vi "find_preamble_2x2.vi"(0 "received \ntime symbol":cdb[][](array[numeric]), 5 "FFT Size":u32, 7 "CP Length":u32, 9 "1st preamble":cdb[](array[numeric]), 11 "2nd preamble":cdb[](array[numeric])) -> (4 "Received OFDM symbol (vector)":cdb[](array[numeric]), 6 "Received OFDM symbol (h11)":cdb[](array[numeric]), 8 "Received OFDM symbol (h12)":cdb[](array[numeric]), 10 "Received OFDM symbol (h21)":cdb[](array[numeric]), 15 "Received OFDM symbol (h22)":cdb[](array[numeric]))   [LabVIEW 2020]
uses:
  <vilib>/Analysis/2dsp.llb/2D Complex FFT.vi
  <vilib>/Analysis/baseanly.llb/Complex A x B.vi
  <vilib>/Analysis/baseanly.llb/Complex Inverse Matrix.vi
  <vilib>/Analysis/baseanly.llb/Complex A x Vector.vi
  <vilib>/Analysis/NI_AALBase.lvlib
  <vilib>/Analysis/NI_AALPro.lvlib
panel:
  out "size(s)":i32
  out "Waveform Chart 4":dbl[][](graph)
  out "Array 2":i32[](array[numeric])
  out "x-y 2":i32
  out "max value 4":dbl
  out "max value 3":dbl
  out "Array":i32[](array[numeric])
  out "x-y":i32
  out "max value 2":dbl
  out "max value":dbl
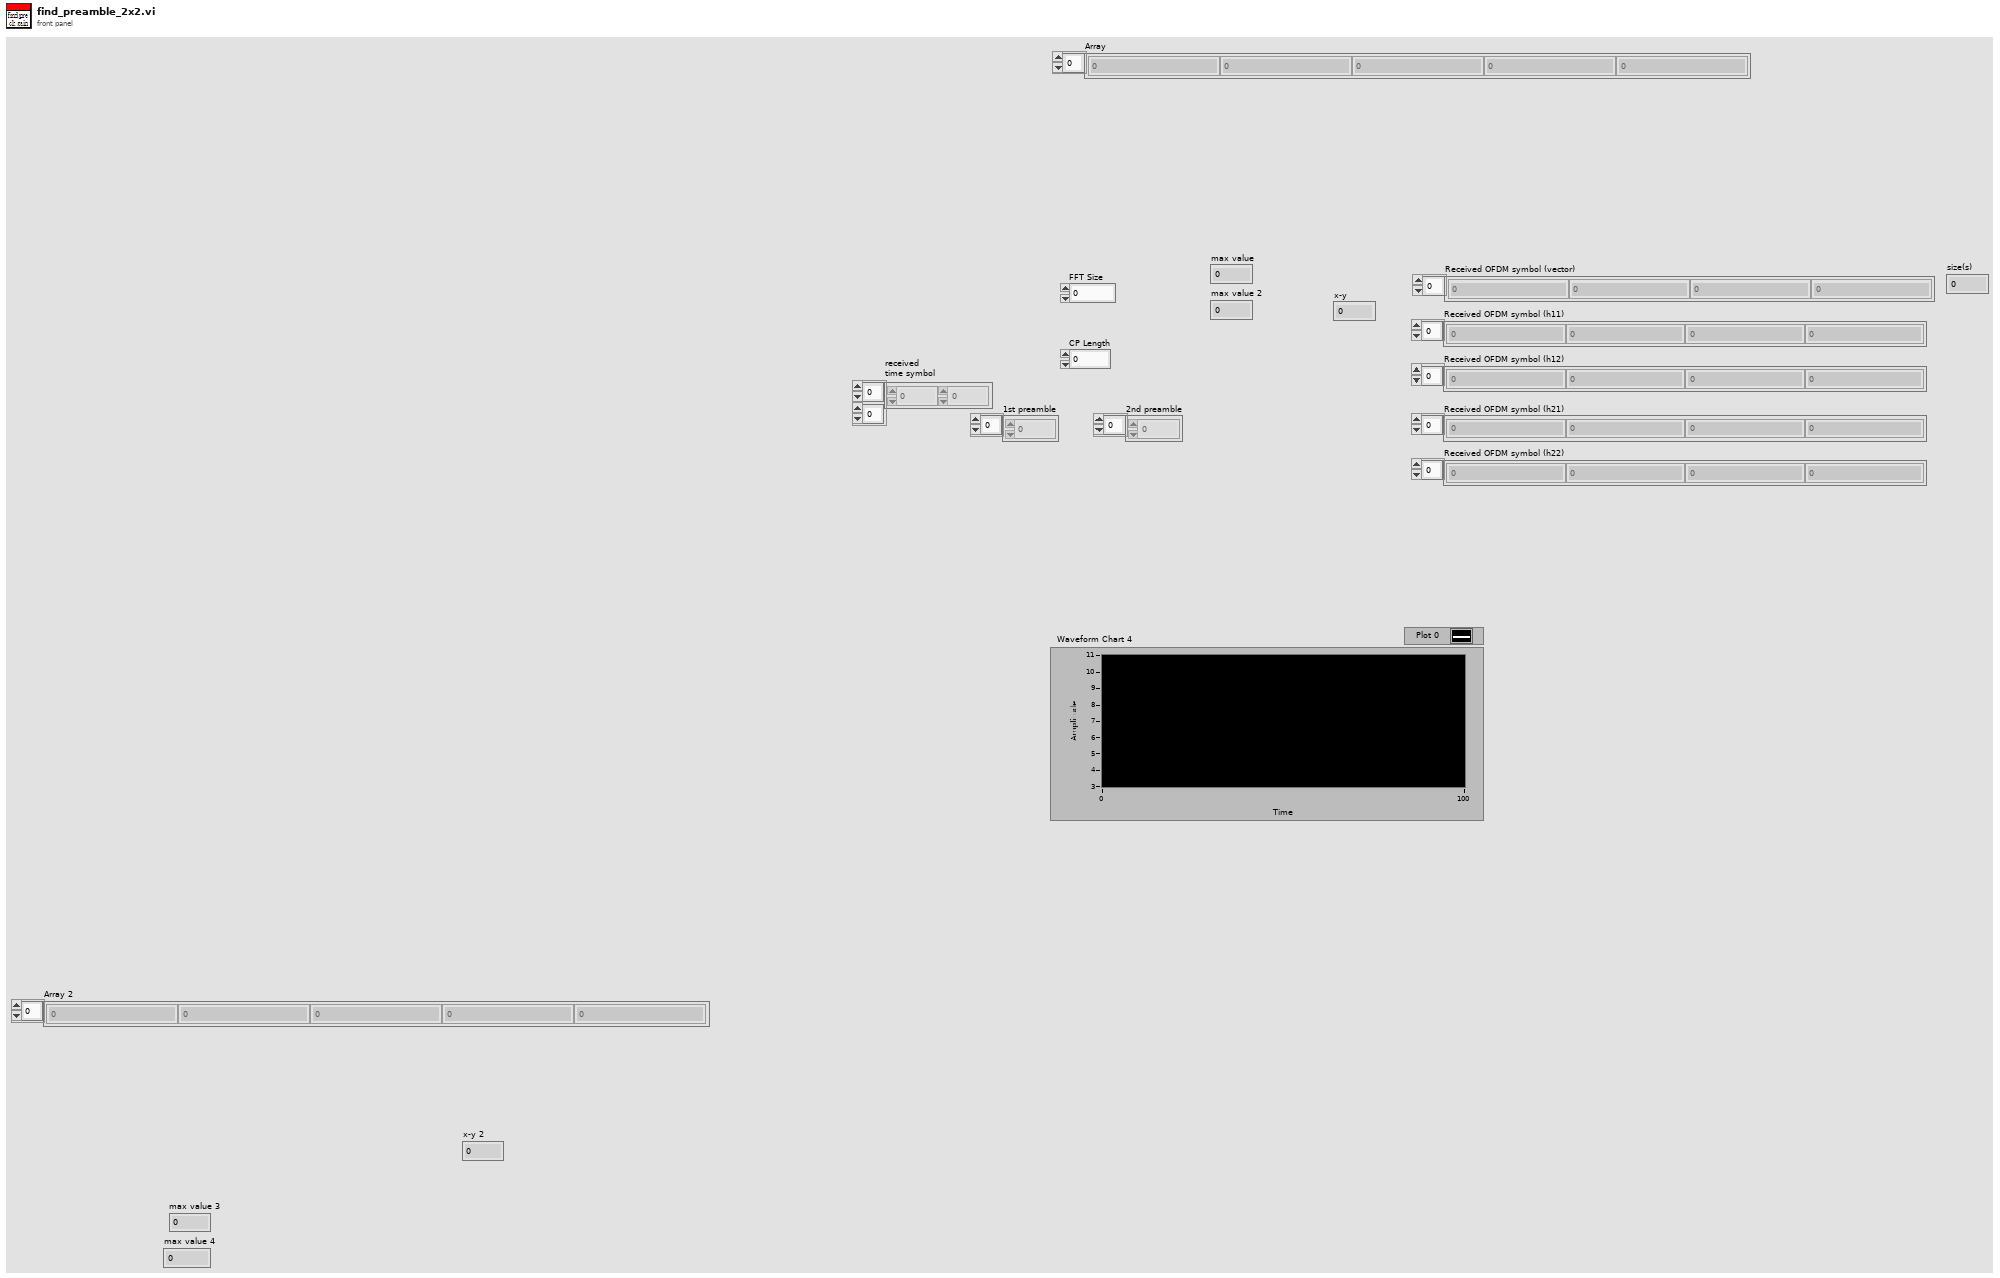
[diagram p1: front panel]
types:
  T1 = typedef "NI_Matrix.lvlib/ComplexMatrix.ctl" = cdb[][]
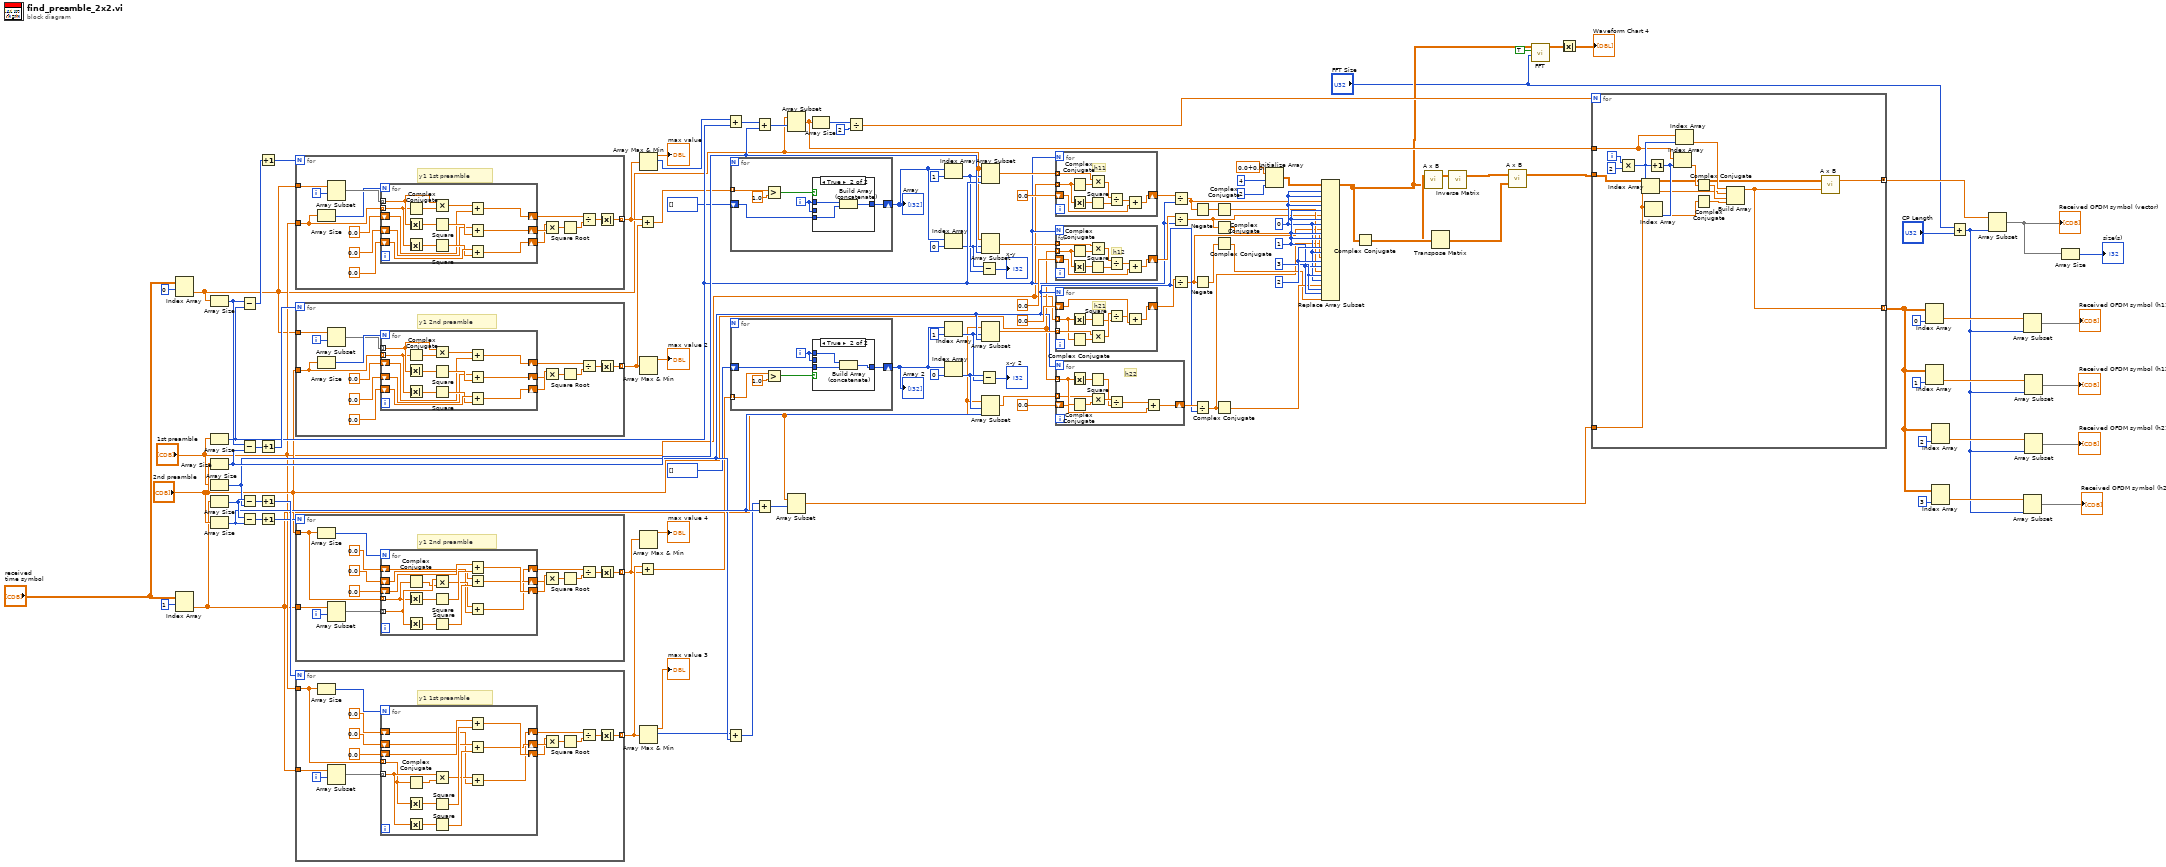
[diagram p0: block diagram]
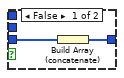
[diagram p2: hidden frame]
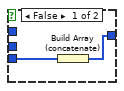
[diagram p3: hidden frame]
diagram:
  w46 = 3
  w47 = 2
  w45 = 1
  w44 = 0
  n1 = Index Array(array="received \ntime symbol", index (row)=0) -> (element=w52:cdb[])  [unwired: 1 in]
  n2 = Index Array(array="received \ntime symbol", index (row)=1) -> (element=w51:cdb[])  [unwired: 1 in]
  n3 = Array Size(array=w52) -> (size(s)=w110:i32)
  n4 = Array Size(array="1st preamble") -> (size(s)=w100:i32)
  n5 = Array Size(array="2nd preamble") -> (size(s)=w102:i32)
  n6 = Array Size(array="1st preamble") -> (size(s)=w72:i32)
  n7 = Array Size(array=w51) -> (size(s)=w80:i32)
  n8 = Array Size(array="2nd preamble") -> (size(s)=w74:i32)
  n9 = Subtract(x=w110, y=w100) -> (x-y=w114:i32)
  n10 = Subtract(x=w110, y=w102) -> (x-y=w112:i32)
  n11 = Subtract(x=w80, y=w72) -> (x-y=w84:i32)
  n12 = Subtract(x=w80, y=w74) -> (x-y=w82:i32)
  n13 = Increment(x=w114) -> (x+1=w113:i32)
  n14 = Increment(x=w112) -> (x+1=w111:i32)
  n15 = Increment(x=w84) -> (x+1=w83:i32)
  n16 = Increment(x=w82) -> (x+1=w81:i32)
  n17 = for {
    N: w113 -> [_]
    tunnel: w52 -> [w117]
    tunnel: "1st preamble" -> [w118]
    tunnel: [w116] -> w93 mode=indexing
    i -> [w115]
    # "y1 1st preamble"
    n18 = Array Size(array=w118) -> (size(s)=w119:i32)
    n19 = Array Subset(array=w117, index=w115) -> (w120:cdb[])  [unwired: 1 in]
    n20 = for {
      N: w119 -> [_]
      tunnel: w118 -> [w130] mode=indexing
      shift-right: [w140] -> w121
      shift-left: 0.0 -> [w142]
      shift-right: [w137] -> w122
      shift-left: 0.0 -> [w136]
      tunnel: w120 -> [w135] mode=indexing
      shift-right: [w131] -> w123
      shift-left: 0.0 -> [w132]
      n21 = Complex Conjugate(1:w130) -> (0:w134:cdb)
      n22 = Absolute Value(x=w135) -> (abs(x)=w139:dbl)
      n23 = Absolute Value(x=w130) -> (abs(x)=w143:dbl)
      n24 = Multiply(x=w135, y=w134) -> (x*y=w133:cdb)
      n25 = Square(x=w139) -> (x^2=w138:dbl)
      n26 = Square(x=w143) -> (x^2=w141:dbl)
      n27 = Add(x=w133, y=w132) -> (x+y=w131:cdb)
      n28 = Add(x=w136, y=w138) -> (x+y=w137:dbl)
      n29 = Add(x=w142, y=w141) -> (x+y=w140:dbl)
    }
    n30 = Multiply(x=w121, y=w122) -> (x*y=w125:dbl)
    n31 = Square Root(x=w125) -> (sqrt(x)=w126:dbl)
    n32 = Divide(x=w123, y=w126) -> (x/y=w124:cdb)
    n33 = Absolute Value(x=w124) -> (abs(x)=w116:dbl)
  }
  n34 = for {
    N: w111 -> [_]
    tunnel: "2nd preamble" -> [w144]
    tunnel: w52 -> [w145]
    tunnel: [w149] -> w92 mode=indexing
    i -> [w152]
    # "y1 2nd preamble"
    n35 = Array Size(array=w144) -> (size(s)=w158:i32)
    n36 = Array Subset(array=w145, index=w152) -> (w157:cdb[])  [unwired: 1 in]
    n37 = for {
      N: w158 -> [_]
      tunnel: w144 -> [w159] mode=indexing
      shift-right: [w169] -> w156
      shift-left: 0.0 -> [w171]
      shift-right: [w166] -> w155
      shift-left: 0.0 -> [w165]
      tunnel: w157 -> [w164] mode=indexing
      shift-right: [w160] -> w154
      shift-left: 0.0 -> [w161]
      n38 = Complex Conjugate(1:w159) -> (0:w163:cdb)
      n39 = Absolute Value(x=w164) -> (abs(x)=w168:dbl)
      n40 = Absolute Value(x=w159) -> (abs(x)=w172:dbl)
      n41 = Multiply(x=w164, y=w163) -> (x*y=w162:cdb)
      n42 = Square(x=w168) -> (x^2=w167:dbl)
      n43 = Square(x=w172) -> (x^2=w170:dbl)
      n44 = Add(x=w162, y=w161) -> (x+y=w160:cdb)
      n45 = Add(x=w165, y=w167) -> (x+y=w166:dbl)
      n46 = Add(x=w171, y=w170) -> (x+y=w169:dbl)
    }
    n47 = Multiply(x=w156, y=w155) -> (x*y=w151:dbl)
    n48 = Square Root(x=w151) -> (sqrt(x)=w150:dbl)
    n49 = Divide(x=w154, y=w150) -> (x/y=w153:cdb)
    n50 = Absolute Value(x=w153) -> (abs(x)=w149:dbl)
  }
  n51 = for {
    N: w81 -> [_]
    tunnel: "2nd preamble" -> [w173]
    tunnel: w51 -> [w174]
    tunnel: [w178] -> w64 mode=indexing
    i -> [w181]
    # "y1 2nd preamble"
    n52 = Array Size(array=w173) -> (size(s)=w187:i32)
    n53 = Array Subset(array=w174, index=w181) -> (w186:cdb[])  [unwired: 1 in]
    n54 = for {
      N: w187 -> [_]
      tunnel: w173 -> [w188] mode=indexing
      shift-right: [w198] -> w185
      shift-left: 0.0 -> [w200]
      shift-right: [w195] -> w184
      shift-left: 0.0 -> [w194]
      tunnel: w186 -> [w193] mode=indexing
      shift-right: [w189] -> w183
      shift-left: 0.0 -> [w190]
      n55 = Complex Conjugate(1:w188) -> (0:w192:cdb)
      n56 = Absolute Value(x=w188) -> (abs(x)=w201:dbl)
      n57 = Absolute Value(x=w193) -> (abs(x)=w197:dbl)
      n58 = Multiply(x=w193, y=w192) -> (x*y=w191:cdb)
      n59 = Square(x=w201) -> (x^2=w199:dbl)
      n60 = Square(x=w197) -> (x^2=w196:dbl)
      n61 = Add(x=w200, y=w199) -> (x+y=w198:dbl)
      n62 = Add(x=w194, y=w196) -> (x+y=w195:dbl)
      n63 = Add(x=w191, y=w190) -> (x+y=w189:cdb)
    }
    n64 = Multiply(x=w185, y=w184) -> (x*y=w180:dbl)
    n65 = Square Root(x=w180) -> (sqrt(x)=w179:dbl)
    n66 = Divide(x=w183, y=w179) -> (x/y=w182:cdb)
    n67 = Absolute Value(x=w182) -> (abs(x)=w178:dbl)
  }
  n68 = for {
    N: w83 -> [_]
    tunnel: w51 -> [w204]
    tunnel: "1st preamble" -> [w205]
    tunnel: [w203] -> w65 mode=indexing
    i -> [w202]
    # "y1 1st preamble"
    n69 = Array Size(array=w205) -> (size(s)=w206:i32)
    n70 = Array Subset(array=w204, index=w202) -> (w207:cdb[])  [unwired: 1 in]
    n71 = for {
      N: w206 -> [_]
      tunnel: w205 -> [w217] mode=indexing
      shift-right: [w227] -> w208
      shift-left: 0.0 -> [w229]
      shift-right: [w224] -> w209
      shift-left: 0.0 -> [w223]
      tunnel: w207 -> [w222] mode=indexing
      shift-right: [w218] -> w210
      shift-left: 0.0 -> [w219]
      n72 = Complex Conjugate(1:w217) -> (0:w221:cdb)
      n73 = Absolute Value(x=w217) -> (abs(x)=w230:dbl)
      n74 = Absolute Value(x=w222) -> (abs(x)=w226:dbl)
      n75 = Multiply(x=w222, y=w221) -> (x*y=w220:cdb)
      n76 = Square(x=w230) -> (x^2=w228:dbl)
      n77 = Square(x=w226) -> (x^2=w225:dbl)
      n78 = Add(x=w229, y=w228) -> (x+y=w227:dbl)
      n79 = Add(x=w223, y=w225) -> (x+y=w224:dbl)
      n80 = Add(x=w220, y=w219) -> (x+y=w218:cdb)
    }
    n81 = Multiply(x=w208, y=w209) -> (x*y=w212:dbl)
    n82 = Square Root(x=w212) -> (sqrt(x)=w213:dbl)
    n83 = Divide(x=w210, y=w213) -> (x/y=w211:cdb)
    n84 = Absolute Value(x=w211) -> (abs(x)=w203:dbl)
  }
  n85 = Add(x=w93, y=w92) -> (x+y=w91:dbl[])
  n86 = Add(x=w65, y=w64) -> (x+y=w63:dbl[])
  n87 = Array Max & Min(array=w93) -> (max value=→"max value":dbl, max index (indices)=w94:i32)  [unwired: 2 out]
  n88 = Array Max & Min(array=w92) -> (max value=→"max value 2":dbl)  [unwired: 3 out]
  n89 = Array Max & Min(array=w64) -> (max value=→"max value 4":dbl)  [unwired: 3 out]
  n90 = Array Max & Min(array=w65) -> (max value=→"max value 3":dbl, max index (indices)=w66:i32)  [unwired: 2 out]
  n91 = Add(x=w94, y=w100) -> (x+y=w101:i32)
  n92 = Add(x=w66, y=w72) -> (x+y=w73:i32)
  n93 = for {
    tunnel: w91 -> [w236] mode=indexing
    shift-right: [w233] -> w88
    shift-left: i32[] [] -> [w232]
    i -> [w231]
    n94 = Greater?(x=w236, y=1.0) -> (0:w234:bool)
    n95 = case shown="True" w234 {
      tunnel: w231 -> [_ _]
      tunnel: [w238 w241] -> w233
      tunnel: w232 -> [w237 w239]
      tunnel: w231 -> [_ w240]
      frame False {
        n96 = Build Array (concatenate)(w237) -> (w238:i32[])
      }
      frame True {
        n97 = Build Array (concatenate)(w240, w239) -> (w241:i32[])
      }
    }
  }
  "Array" <- w88
  n98 = for {
    tunnel: w63 -> [w247] mode=indexing
    shift-right: [w244] -> w60
    shift-left: i32[] [] -> [w243]
    i -> [w242]
    n99 = Greater?(x=w247, y=1.0) -> (0:w245:bool)
    n100 = case shown="True" w245 {
      tunnel: w242 -> [_ _]
      tunnel: [w249 w252] -> w244
      tunnel: w243 -> [w248 w250]
      tunnel: w242 -> [_ w251]
      frame False {
        n101 = Build Array (concatenate)(w248) -> (w249:i32[])
      }
      frame True {
        n102 = Build Array (concatenate)(w251, w250) -> (w252:i32[])
      }
    }
  }
  "Array 2" <- w60
  n103 = Add(x=w101, y=w102) -> (x+y=w99:i32)
  n104 = Add(x=w73, y=w74) -> (x+y=w71:i32)
  n105 = Array Subset(array=w52, index=w99) -> (w28:cdb[])  [unwired: 1 in]
  n106 = Array Subset(array=w51, index=w71) -> (w27:cdb[])  [unwired: 1 in]
  n107 = Array Size(array=w28) -> (size(s)=w109:i32)
  n108 = Divide(x=w109, y=2) -> (x/y=w26:dbl)
  n109 = Index Array(array=w88, index=1) -> (element=w85:i32)
  n110 = Index Array(array=w88, index=0) -> (element=w86:i32)
  n111 = Index Array(array=w60, index=1) -> (element=w57:i32)
  n112 = Index Array(array=w60, index=0) -> (element=w58:i32)
  n113 = Subtract(x=w86, y=w85) -> (x-y=→"x-y":i32)
  n114 = Subtract(x=w58, y=w57) -> (x-y=→"x-y 2":i32)
  n115 = Array Subset(array=w52, index=w85, length=w100) -> (w103:cdb[])
  n116 = Array Subset(array=w52, index=w86, length=w102) -> (w98:cdb[])
  n117 = Array Subset(array=w51, index=w57, length=w72) -> (w75:cdb[])
  n118 = Array Subset(array=w51, index=w58, length=w74) -> (w70:cdb[])
  n119 = for {
    N: w100 -> [_]
    shift-right: [w254] -> w107
    shift-left: 0.0 -> [w256]
    tunnel: w103 -> [w259] mode=indexing
    tunnel: "1st preamble" -> [w253] mode=indexing
    # "h11"
    n120 = Complex Conjugate(1:w253) -> (0:w261:cdb)
    n121 = Absolute Value(x=w253) -> (abs(x)=w260:dbl)
    n122 = Square(x=w260) -> (x^2=w257:dbl)
    n123 = Multiply(x=w259, y=w261) -> (x*y=w258:cdb)
    n124 = Divide(x=w258, y=w257) -> (x/y=w255:cdb)
    n125 = Add(x=w255, y=w256) -> (x+y=w254:cdb)
  }
  n126 = for {
    N: w100 -> [_]
    shift-right: [w264] -> w105
    shift-left: 0.0 -> [w266]
    tunnel: "2nd preamble" -> [w263] mode=indexing
    tunnel: w98 -> [w262] mode=indexing
    # "h12"
    n127 = Complex Conjugate(1:w263) -> (0:w270:cdb)
    n128 = Absolute Value(x=w263) -> (abs(x)=w269:dbl)
    n129 = Square(x=w269) -> (x^2=w267:dbl)
    n130 = Multiply(x=w262, y=w270) -> (x*y=w268:cdb)
    n131 = Divide(x=w268, y=w267) -> (x/y=w265:cdb)
    n132 = Add(x=w265, y=w266) -> (x+y=w264:cdb)
  }
  n133 = for {
    N: w72 -> [_]
    shift-right: [w272] -> w79
    shift-left: 0.0 -> [w274]
    tunnel: w75 -> [w277] mode=indexing
    tunnel: "1st preamble" -> [w271] mode=indexing
    # "h21"
    n134 = Absolute Value(x=w271) -> (abs(x)=w278:dbl)
    n135 = Complex Conjugate(1:w271) -> (0:w279:cdb)
    n136 = Square(x=w278) -> (x^2=w275:dbl)
    n137 = Multiply(x=w277, y=w279) -> (x*y=w276:cdb)
    n138 = Divide(x=w276, y=w275) -> (x/y=w273:cdb)
    n139 = Add(x=w273, y=w274) -> (x+y=w272:cdb)
  }
  n140 = for {
    N: w72 -> [_]
    shift-right: [w282] -> w77
    shift-left: 0.0 -> [w284]
    tunnel: "2nd preamble" -> [w281] mode=indexing
    tunnel: w70 -> [w280] mode=indexing
    # "h22"
    n141 = Absolute Value(x=w281) -> (abs(x)=w287:dbl)
    n142 = Complex Conjugate(1:w281) -> (0:w288:cdb)
    n143 = Square(x=w287) -> (x^2=w285:dbl)
    n144 = Multiply(x=w280, y=w288) -> (x*y=w286:cdb)
    n145 = Divide(x=w286, y=w285) -> (x/y=w283:cdb)
    n146 = Add(x=w283, y=w284) -> (x+y=w282:cdb)
  }
  n147 = Divide(x=w107, y=w100) -> (x/y=w31:cdb)
  n148 = Divide(x=w105, y=w100) -> (x/y=w32:cdb)
  n149 = Divide(x=w79, y=w72) -> (x/y=w29:cdb)
  n150 = Negate(x=w31) -> (-x=w34:cdb)
  n151 = Negate(x=w29) -> (-x=w33:cdb)
  n152 = Divide(x=w77, y=w72) -> (x/y=w30:cdb)
  n153 = Complex Conjugate(1:w34) -> (0:w37:cdb)
  n154 = Complex Conjugate(1:w32) -> (0:w38:cdb)
  n155 = Complex Conjugate(1:w33) -> (0:w35:cdb)
  n156 = Complex Conjugate(1:w30) -> (0:w36:cdb)
  n157 = Initialize Array(cdb 0.0+0.0i, 4, 2) -> (w48:cdb[][])
  n158 = Replace Array Subset(array=w48, new element #1=w31, index (row) #1=w44, index (col) #1=w44, new element #2=w32, index (row) #2=w44, index (col) #2=w45, new element #3=w29, index (row) #3=w45, index (col) #3=w44, new element #4=w30, index (row) #4=w45, index (col) #4=w45, new element #5=w38, index (row) #5=w47, index (col) #5=w44, new element #6=w37, index (row) #6=w47, index (col) #6=w45, new element #7=w36, index (row) #7=w46, index (col) #7=w44, new element #8=w35, index (row) #8=w46, index (col) #8=w45) -> (w19:cdb[][])
  n159 = Complex Conjugate(1:w19) -> (0:w42:cdb[][])
  n160 = Transpose Matrix(1:w42) -> (0:w40:cdb[][])
  n161 = call-poly <vilib>:"A x B.vi"("B"=w19, "A"=w40) -> ("A x B"=w41:T1)  [unwired: 1 out]
  n162 = call-poly <vilib>:"Inverse Matrix.vi"("Input Matrix"=w41) -> ("Inverse Matrix"=w39:T1)  [unwired: 1 in, 1 out]
  n163 = call-poly <vilib>:"A x B.vi"("B"=w40, "A"=w39) -> ("A x B"=w20:T1)  [unwired: 1 out]
  n164 = call-poly <vilib>:"FFT.vi"("m"="FFT Size", "shift?"=TRUE, "X"=w19) -> ("FFT {X}"=w22:cdb[][])  [unwired: 7 in, 1 out]
  n165 = Absolute Value(x=w22) -> (abs(x)=→"Waveform Chart 4":dbl[][])
  n166 = for {
    N: w26 -> [_]
    tunnel: w20 -> [w291]
    tunnel: [w290] -> w25 mode=concatenating
    tunnel: w28 -> [w297]
    tunnel: w27 -> [w296]
    tunnel: [w289] -> w10 mode=indexing
    i -> [w303]
    n167 = Multiply(x=w303, y=2) -> (x*y=w301:i32)
    n168 = Index Array(array=w296, index=w301) -> (element=w294:cdb)
    n169 = Increment(x=w301) -> (x+1=w300:i32)
    n170 = Index Array(array=w296, index=w300) -> (element=w292:cdb)
    n171 = Index Array(array=w297, index=w300) -> (element=w293:cdb)
    n172 = Index Array(array=w297, index=w301) -> (element=w295:cdb)
    n173 = Complex Conjugate(1:w293) -> (0:w299:cdb)
    n174 = Complex Conjugate(1:w292) -> (0:w298:cdb)
    n175 = Build Array "Build Array"(w295, w294, w299, w298) -> (w289:cdb[])
    n176 = call-poly <vilib>:"A x B.vi"("Vector"=w289, "A"=w291) -> ("A x Vector"=w290:cdb[])  [unwired: 1 out]
  }
  n177 = Index Array(array=w10, index (col)=0 ("disabled index (col)")) -> (element=w11:cdb[])  [unwired: 1 in]
  n178 = Index Array(array=w10, index (col)=1 ("disabled index (col)")) -> (element=w9:cdb[])  [unwired: 1 in]
  n179 = Index Array(array=w10, index (col)=2 ("disabled index (col)")) -> (element=w8:cdb[])  [unwired: 1 in]
  n180 = Index Array(array=w10, index (col)=3 ("disabled index (col)")) -> (element=w7:cdb[])  [unwired: 1 in]
  n181 = Add(x="FFT Size", y="CP Length") -> (x+y=w6:u32)
  n182 = Array Subset "Array Subset"(array=w25, length=w6) -> (w24:cdb[])  [unwired: 1 in]
  "Received OFDM symbol (vector)" <- w24
  n183 = Array Subset "Array Subset"(array=w11, length=w6) -> (→"Received OFDM symbol (h11)":cdb[])  [unwired: 1 in]
  n184 = Array Subset "Array Subset"(array=w7, length=w6) -> (→"Received OFDM symbol (h22)":cdb[])  [unwired: 1 in]
  n185 = Array Subset "Array Subset"(array=w9, length=w6) -> (→"Received OFDM symbol (h12)":cdb[])  [unwired: 1 in]
  n186 = Array Subset "Array Subset"(array=w8, length=w6) -> (→"Received OFDM symbol (h21)":cdb[])  [unwired: 1 in]
  n187 = Array Size(array=w24) -> (size(s)=→"size(s)":i32)
